vi "navX Close.vi"(0 "navX Device":T1={"Interface"={"Protocol"=enum."SERIAL", "Update Rate (4Hz-60Hz)"=4, "navX Open TypeDef"=variant}, "Notifiy Packet"=refnum, "Loop VI Refnum"=refnum} {"Interface"."Update Rate (4Hz-60Hz)" min=4 max=60 step=1}) -> ()   [LabVIEW 2014, in "navX Library v2.lvlib"]
uses:
  navX Library v2.lvlib
  TypeDefs/navX Device TypeDef.ctl
  TypeDefs/navX Protocol TypeDef.ctl
  TypeDefs/navX Notify Packet TypeDef.ctl
  TypeDefs/navX Action TypeDef.ctl
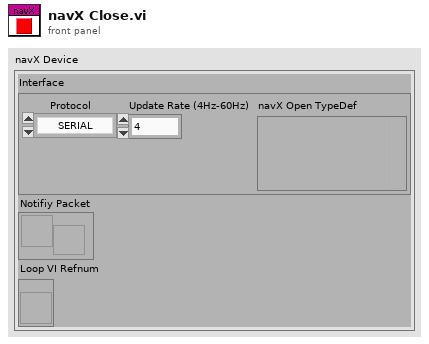
[diagram p1: front panel]
types:
  T1 = typedef "navX Library v2.lvlib/navX Device TypeDef.ctl" = cluster{"Interface":cluster{"Protocol":T2, "Update Rate (4Hz-60Hz)":u8, "navX Open TypeDef":variant}, "Notifiy Packet":refnum<notifier>, "Loop VI Refnum":refnum<vi>}
  T2 = typedef "navX Library v2.lvlib/navX Protocol TypeDef.ctl" = enum16{"SERIAL", "I2C", "SPI"}
  T3 = typedef "navX Library v2.lvlib/navX Notify Packet TypeDef.ctl" = cluster{"navX Action":T4, "Data":variant}
  T4 = typedef "navX Library v2.lvlib/navX Action TypeDef.ctl" = enum16{"None", "Halt", "Reboot Detected", "Zero-Yaw"}
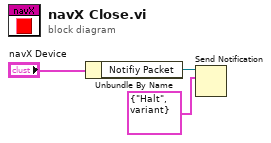
[diagram p0: block diagram]
diagram:
  n1 = Unbundle By Name("navX Device") -> ("Notifiy Packet"=w2:refnum<notifier>)
  n2 = Send Notification(notification=T3 {"navX Action"=enum."Halt", "Data"=variant}, notifier=w2) -> ()  [unwired: 1 in, 2 out]
